vi "qKLS.vi"(0 "System no.":i32=1 min=1 max=4 step=1, 2 "Name":string, 5 "error in":errorcluster, 6 "Item":string, 7 "Item 2":string) -> (14 "Response":string, 19 "error out":errorcluster)   [LabVIEW 2026]
doc: "Returns parameters of all available coordinate systems. The returned information depends on the used arguments. To query parameters of Work/Tool combinations use the KLC? Command. The x, y, z, u, v, w values of all levelling coordinate systems are displayed according to current coordinate system settings. Item is only valid in combination with Name; Item 2 is only valid in combination with Name and Item.\n\nC-887, F-206, M-8X0: Only for GCS syntax version = GCS 2.0 or higher (Check with CSV?.vi. If CSV?.vi is not supported, syntax version is GCS 1.0)."
panel:
  # "Returns parameters of all available coordinate systems. \nThe returned information depends on the used arguments."
  # "Only valid in combination\nwith Name:"
  # "Only valid in combination\nwith Name + Item:"
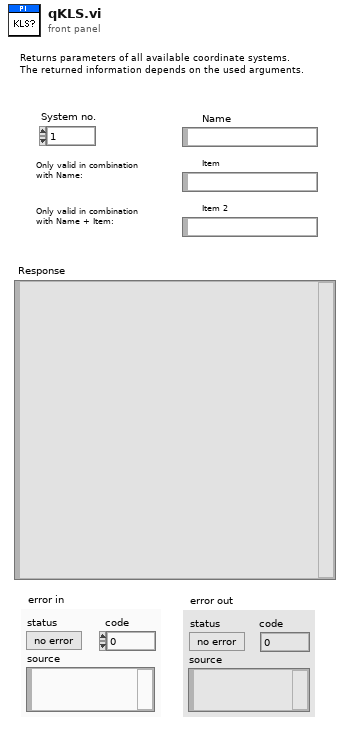
[diagram p1: front panel]
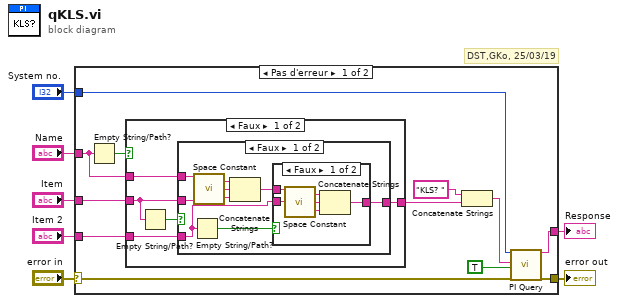
[diagram p0: block diagram]
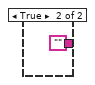
[diagram p4: hidden frame]
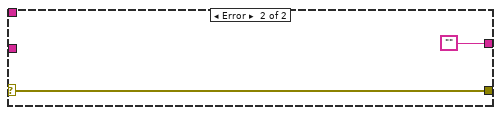
[diagram p5: hidden frame]
diagram:
  # "DST,GKo, 25/03/19"
  n1 = case shown="Pas d'erreur" "error in" {
    selector: "error in" -> [w12 w40]
    tunnel: [w11 ""] -> w7
    tunnel: [w10 w40] -> w6
    tunnel: "System no." -> [w19 _]
    tunnel: "Name" -> [w8 _]
    tunnel: "Item" -> [w16 _]
    tunnel: "Item 2" -> [w15 _]
    frame No Error {
      n2 = Empty String/Path?(string/path=w8) -> (empty?=w9:bool)
      n3 = case shown="Faux" w9 {
        tunnel: w16 -> [w20 _]
        tunnel: w15 -> [w24 _]
        tunnel: [w23 ""] -> w14
        tunnel: w8 -> [w22 _]
        frame False {
          n4 = Empty String/Path?(string/path=w20) -> (empty?=w21:bool)
          n5 = case shown="Faux" w21 {
            tunnel: w24 -> [w26 _]
            tunnel: [w31 w37] -> w23
            tunnel: w22 -> [w30 w37]
            tunnel: w20 -> [w27 _]
            frame False {
              n6 = Empty String/Path?(string/path=w26) -> (empty?=w25:bool)
              n7 = call <vilib>:"Space Constant.vi"() -> ("String"=w28:string)
              n8 = Concatenate Strings(w30, w28, w27) -> (w29:string)
              n9 = case shown="Faux" w25 {
                tunnel: [w32 w36] -> w31
                tunnel: w29 -> [w35 w36]
                tunnel: w26 -> [w33 _]
                frame False {
                  n10 = call <vilib>:"Space Constant.vi"() -> ("String"=w34:string)
                  n11 = Concatenate Strings(w35, w34, w33) -> (w32:string)
                }
                frame True {
                }
              }
            }
            frame True {
            }
          }
        }
        frame True {
        }
      }
      n12 = Concatenate Strings("KLS? " ("string"), w14) -> (w17:string)
      n13 = call "PI Query.vi"("System no."=w19, "String to send"=w17, "Attach termination char.?"=TRUE ("Attach Linefeed?"), "error in"=w12) -> ("String read"=w11:string, "error out"=w10:errorcluster)  [unwired: 3 in, 11 out]
    }
    frame Error {
    }
  }
  "Response" <- w7
  "error out" <- w6
